vi "Tree Set Current.vi"(8 "error in (no error)":errorcluster, 9 "Shot":i32, 10 "Tree name":string, 11 "Tree DVR in":refnum<data-value>) -> (0 "error out":errorcluster, 3 "Tree DVR out":refnum<data-value>)   [LabVIEW 2010, in "MDSplus.lvlib"]
doc: "Set the current tree and shot."
uses:
  <vilib>/MDSplus/Library/MDSplus.lvlib
  <vilib>/MDSplus/Classes/Tree_Class/Tree.lvclass
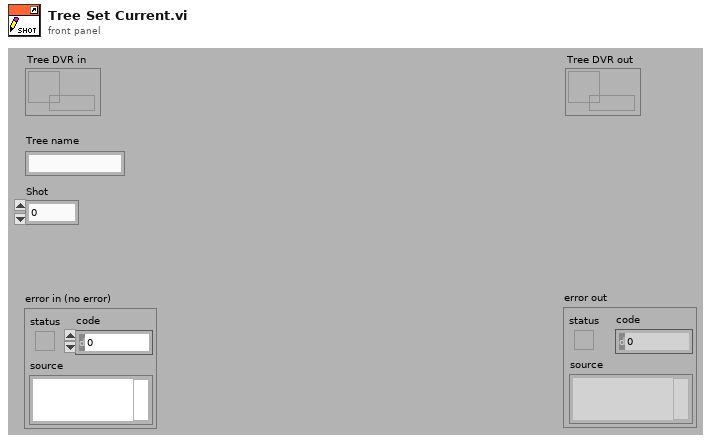
[diagram p1: front panel]
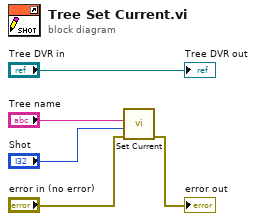
[diagram p0: block diagram]
diagram:
  n1 = call <vilib>:"Set Current.vi"("error in (no error)"="error in (no error)", "Shot"="Shot", "Tree name"="Tree name") -> ("error out"=→"error out":errorcluster)  [unwired: 7 in, 1 out]
  "Tree DVR out" <- "Tree DVR in"
